vi "Get IConfiguration.vi"(11 "gRPC XNET Read Raw CAN Frame in":refnum<class "gRPC XNET Read Raw CAN Frame Strategy.lvclass">) -> (2 "IConfiguration":refnum<class "IConfiguration.lvclass">, 3 "gRPC XNET Read Raw CAN Frame out":refnum<class "gRPC XNET Read Raw CAN Frame Strategy.lvclass">)   [LabVIEW 2024, in "gRPC XNET Read Raw CAN Frame Strategy.lvclass"]
uses:
  gRPC XNET Read Raw CAN Frame Strategy.lvclass
  gRPC XNET Read Raw CAN Frame Strategy.lvclass/gRPC XNET Read Raw CAN Frame Strategy.ctl
  Source/Interfaces/IConfiguration/IConfiguration.lvclass
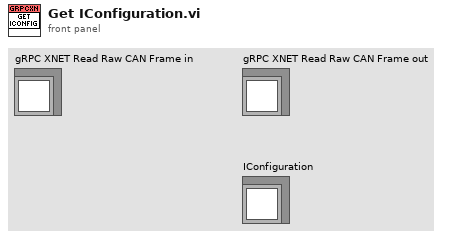
[diagram p1: front panel]
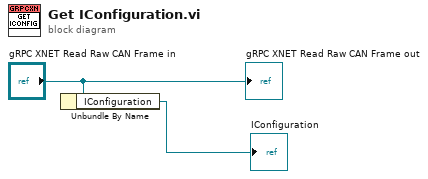
[diagram p0: block diagram]
diagram:
  n1 = Unbundle By Name("gRPC XNET Read Raw CAN Frame in") -> ("IConfiguration"=→"IConfiguration":refnum<class "IConfiguration.lvclass">)
  "gRPC XNET Read Raw CAN Frame out" <- "gRPC XNET Read Raw CAN Frame in"
